vi "onCreated.vi"(8 "error in (no error)":errorcluster, 11 "Microscope":refnum<class "Microscope.lvclass">) -> (0 "error out":errorcluster, 3 "Microscope out":refnum<class "Microscope.lvclass">)   [LabVIEW 2015, in "Microscope.lvclass"]
doc: "JKI State Machine Objects (SMO) 1.0.4.18\nJKI - JKI\nCopyright (c) 2016, JKI"
uses:
  Microscope.lvclass
  Typedefs/Configuration--Cluster.ctl
  <vilib>/JKI/JKI SMO/SMO/SMO.lvclass
  <vilib>/Utility/config.llb/NI_LVConfig.lvlib
panel:
  # "For instructions on how to use the JKI State Machine Objects, examples and video tutorials, visit:\nhttp://jki.net/state-machine-objects/\n\nJKI State Machine Objects™\nhttp://jki.net/state-machine-objects/\nCopyright (C) 2005-2015, JKI <info@jki.net>\nALL RIGHTS RESERVED"
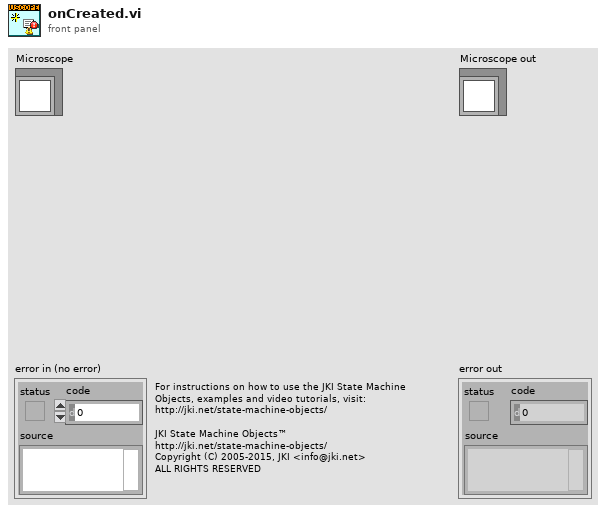
[diagram p1: front panel]
types:
  T1 = typedef "Microscope.lvclass/Configuration--Cluster.ctl" = cluster{"XY Stage":string, "Camera":string, "image output folder":path, "filetype":string}
  T2 = typedef "NI_LVConfig.lvlib/Config Data RefNum.ctl" = refnum<k1>
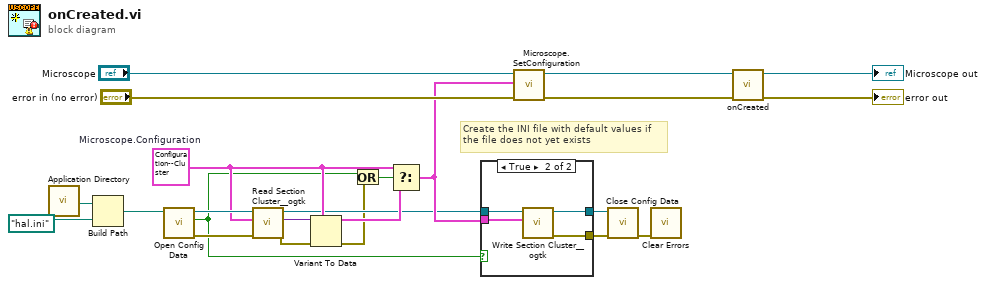
[diagram p0: block diagram]
diagram:
  w11 = T1 {"XY Stage"="Simulated", "Camera"="Simulated", "image output folder"=path "", "filetype"="png"}  # Microscope.Configuration
  # "Create the INI file with default values if\nthe file does not yet exists"
  n1 = call <vilib>:"Application Directory.vi"() -> ("Application Directory"=w19:path)
  n2 = Build Path(base path=w19, name or relative path=path "hal.ini") -> (appended path=w13:path)
  n3 = call <vilib>:"Open Config Data.vi"("configuration file path"=w13) -> ("error out"=w9:errorcluster, "file created?"=w2:bool, "refnum"=w12:T2)  [unwired: 8 in]
  n4 = call <userlib>:"Read Section Cluster__ogtk.vi"("error in (no error)"=w9, "Section Formatted Cluster Type"=w11, "refnum"=w12) -> ("error out"=w4:errorcluster, "Section Formatted Cluster"=w10:variant, "dup refnum"=w8:T2)  [unwired: 4 in, 2 out]
  n5 = Variant To Data(error in=w4, type=w11, Variant=w10) -> (data=w17:T1, error out=w3:errorcluster)
  n6 = Or(x=w2, y=w3) -> (x .or. y?=w1:bool)
  n7 = Select(t=w11, s=w1, f=w17) -> (s? t:f=w16:T1)
  n8 = case shown="True" w2 {
    tunnel: w8 -> [w24 w28]
    tunnel: w16 -> [_ w27]
    tunnel: [_ w26] -> w7
    tunnel: [w24 w25] -> w6
    frame False {
    }
    frame True {
      n9 = call <userlib>:"Write Section Cluster__ogtk.vi"("Section Formatted Cluster"=w27, "refnum"=w28) -> ("error out"=w26:errorcluster, "dup refnum"=w25:T2)  [unwired: 8 in]
    }
  }
  n10 = call "Microscope.SetConfiguration.vi"("error in (no error)"="error in (no error)", "Configuration"=w16, "Microscope"="Microscope") -> ("error out"=w20:errorcluster, "Microscope out"=w22:refnum<class "Microscope.lvclass">)  [unwired: 7 in]
  n11 = call <vilib>:"Close Config Data.vi"("error in (no error)"=w7, "refnum"=w6) -> ("error out"=w5:errorcluster)  [unwired: 8 in, 1 out]
  n12 = call <vilib>:"Clear Errors.vi"("error in (no error)"=w5) -> ()  [unwired: 5 in, 2 out]
  n13 = call-parent "onCreated.vi"("error in (no error)"=w20, "SMO"=w22) -> ("error out"=→"error out":errorcluster, "SMO out"=→"Microscope out":refnum<class "Microscope.lvclass">)  [unwired: 8 in]
